vi "Discovery Endpoint.vi"(8 "error in (no error)":errorcluster, 11 "Cluster in":refnum<class "Cluster Config.lvclass">) -> (0 "error out":errorcluster, 2 "Discovery Endpoint":T1, 3 "Cluster out":refnum<class "Cluster Config.lvclass">)   [LabVIEW 2020, in "VolatusConfig.lvlib" / "Cluster Config.lvclass"]
uses:
  Cluster Config.lvclass
  C:/dev/lv20CE/relink/lv-volatus/VolatusConfig/VolatusConfigElement/VolatusConfigElement.lvclass
  VolatusConfigElement/VolatusConfigElement.lvclass/VolatusConfigElement.ctl
  VolatusConfigElement/Element.vi
  Cluster Config.lvclass/Cluster Config.ctl
  VolatusConfigElement/VolatusConfigElement.lvclass
  lv-cdm/CDM-Config/Config Element/Config Element.lvclass
  lv-vecto/VectoConfig/Endpoint.ctl
  lv-vecto/VectoConfig/VectoConfig.lvlib
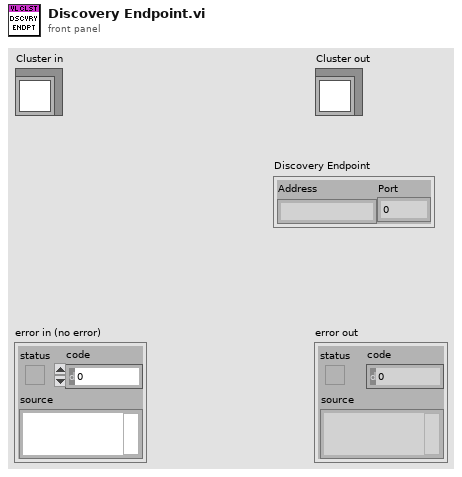
[diagram p1: front panel]
types:
  T1 = typedef "VectoConfig.lvlib/Endpoint.ctl" = cluster{"Address":string, "Port":u16}
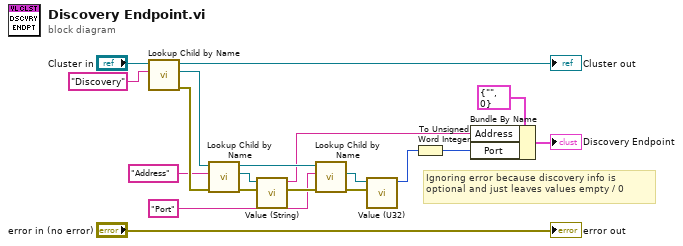
[diagram p0: block diagram]
diagram:
  # "Ignoring error because discovery info is optional and just leaves values empty / 0"
  n1 = call "Lookup Child by Name.vi"("Child Name"="Discovery", "VolatusConfigElement in"="Cluster in") -> ("error out"=w19:errorcluster, "Child"=w12:refnum<class "Config Element.lvclass">, "VolatusConfigElement out"=→"Cluster out":refnum<class "Cluster Config.lvclass">)  [unwired: 6 in, 1 out]
  n2 = call "Lookup Child by Name.vi"("error in (no error)"=w19, "Name"="Address", "Config Element in"=w12) -> ("error out"=w9:errorcluster, "Child"=w10:refnum<class "Config Element.lvclass">, "Config Element out"=w8:refnum<class "Config Element.lvclass">)  [unwired: 5 in, 1 out]
  n3 = call "Value (String).vi"("error in (no error)"=w9, "Config Element in"=w10) -> ("error out"=w6:errorcluster, "String Value"=w7:string)  [unwired: 8 in]
  n4 = call "Lookup Child by Name.vi"("error in (no error)"=w6, "Name"="Port", "Config Element in"=w8) -> ("error out"=w5:errorcluster, "Child"=w4:refnum<class "Config Element.lvclass">)  [unwired: 5 in, 2 out]
  n5 = call "Value (U32).vi"("error in (no error)"=w5, "Config Element in"=w4) -> ("U32 Value"=w3:u32)  [unwired: 8 in, 1 out]
  n6 = To Unsigned Word Integer(number=w3) -> (unsigned 16bit integer=w2:u16)
  n7 = Bundle By Name(cluster=T1 {"Address"="", "Port"=0} ("Discovery Endpoint"), "Address"=w7, "Port"=w2) -> (→"Discovery Endpoint":T1)
  "error out" <- "error in (no error)"
